vi "PDC_SetTriggerMode.vi"(0 "DeviceNo":u32, 5 "Mode":u32, 7 "AFrames":u32, 9 "RFrames":u32, 11 "error in (no error)":errorcluster, 12 "RCount":u32) -> (4 "ReturnValue":u32, 14 "ErrorCode":u32, 15 "error out":errorcluster)   [LabVIEW 2015]
doc: "This VI sets the trigger mode of the specified device."
uses:
  PDCLIB.dll
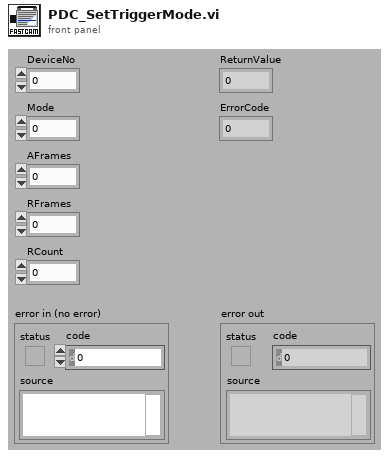
[diagram p1: front panel]
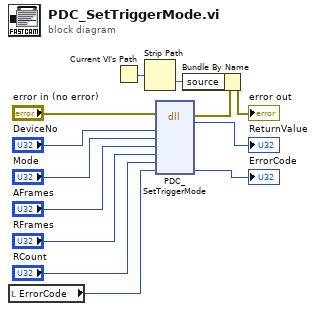
[diagram p0: block diagram]
diagram:
  n1 = local read "ErrorCode"() -> (w10:u32)
  n2 = Current VI's Path() -> (path=w3:path)
  n3 = Strip Path(path=w3) -> (name=w4:string)  [unwired: 1 out]
  n4 = dll-call lib="PDCLIB.dll" fn="PDC_SetTriggerMode"(error in="error in (no error)", "nDeviceNo"="DeviceNo", "nMode"="Mode", "nAFrames"="AFrames", "nRFrames"="RFrames", "nRCount"="RCount", "pErrorCode"=w10) -> (error out=w2:errorcluster, "return type"=→"ReturnValue":u32, "pErrorCode"=→"ErrorCode":u32)  [unwired: 7 in, 1 out]
  n5 = Bundle By Name(cluster=w2, "source"=w4) -> (→"error out":errorcluster)
